vi "Main.vi"() -> ()   [LabVIEW 2014]
doc: "This template is for the Queued Message Handler design pattern.\n\nThe Event Handling Loop generates messages based on user interface actions.\n\nThe Message Handling Loop processes messages generated by the Event Handling Loop, or by other messages. The messages are string values, so new messages can be added easily to the Message Cases case structure in the Message Handling Loop. Each message cluster can also provide an optional value for Message Data, which is a variant that can be converted to whatever message-specific data is required."
uses:
  controls/MHL Data.ctl
  controls/MHL UI Data.ctl
  controls/MHL Status.ctl
  controls/MHL References.ctl
  controls/MHL Configuration.ctl
  support/Boiler System Globals.vi
  support/Message Queue/Message Queue.lvlib
  support/User Event - Stop/User Event - Stop.lvlib
  Boiler/Boiler.lvlib
panel:
  in  "Fuel Control Valve":u32(slide) scale=10.0..75.0
  in  "Stop Boiler":bool
  in  "Light Pilot":bool
  out "Forced Draft Fan":bool
  out "Pilot":bool
  out "Pilot Gas Valve":bool
  out "Primary Fan":bool
  out "Status":string
  in  "Start":bool
  in  "Reset":bool
  in  "Emergency Stop":bool
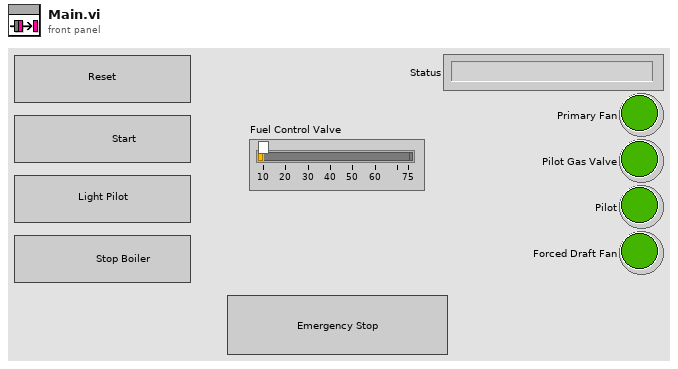
[diagram p1: front panel]
types:
  T1 = typedef "MHL Data.ctl" = cluster{"MHL User Interface Data":T2, "MHL References":T4, "MHL Configuration":T5}
  T2 = typedef "MHL UI Data.ctl" = cluster{"Status":string, "Fuel Control Valve":u32, "Primary Fan":bool, "Pilot Gas Valve":bool, "Pilot":bool, "Forced Draft Fan":bool, "MHL Status":T3}
  T3 = typedef "MHL Status.ctl" = enum16{"Lockout", "Ready", "Pre-Purge", "Pre-Purge Complete", "Pilot On", "Boiler Running", "Shutdown", "Purge"}
  T4 = typedef "MHL References.ctl" = cluster{"Reset Ref":refnum<vi>, "Start Ref":refnum<vi>, "Light Pilot Ref":refnum<vi>, "Stop Boiler Ref":refnum<vi>, "Fuel Control Valve Ref":refnum<vi>}
  T5 = typedef "MHL Configuration.ctl" = cluster{"Fuel Control Valve Maximum":dbl, "Fuel Control Valve Minimum":dbl}
  T6 = typedef "Notifiers.ctl" = cluster{"Handshake":refnum<notifier>, "Flame Level":refnum<notifier>, "Controller Exit":refnum<notifier>, "Boiler Exit":refnum<notifier>}
  T7 = typedef "Message Queue.lvlib/All Message Queues.ctl" = cluster{"MHL":refnum<queue>, "Boiler Controller":refnum<queue>, "Boiler":refnum<queue>}
  T8 = enum32{"invalid app kind", "Development System", "Run Time System", "Student Edition", "Embedded LabVIEW", "Evaluation", "Custom"}
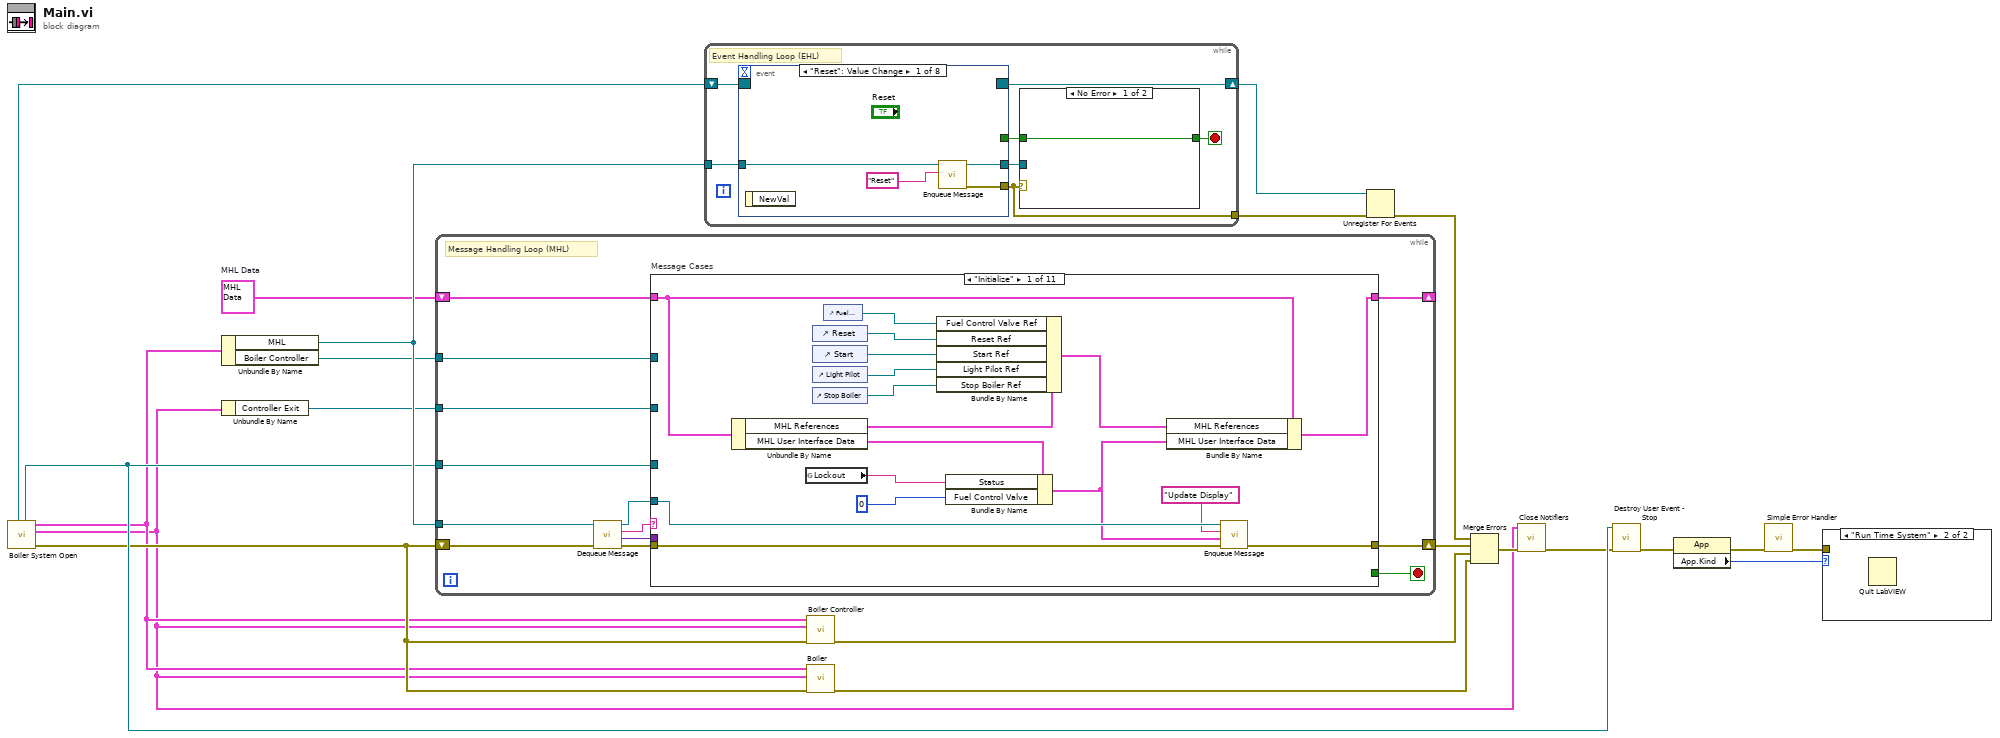
[diagram p0: block diagram]
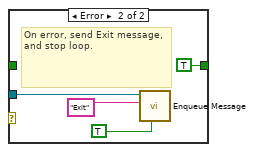
[diagram p3: hidden frame]
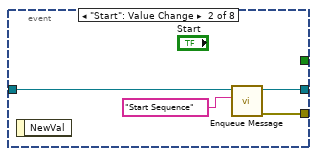
[diagram p4: hidden frame]
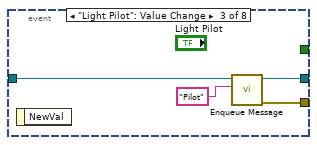
[diagram p5: hidden frame]
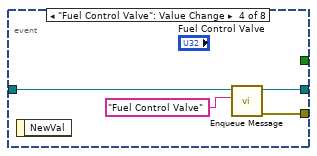
[diagram p6: hidden frame]
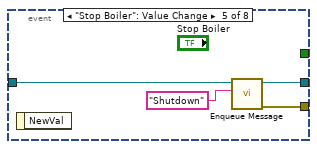
[diagram p7: hidden frame]
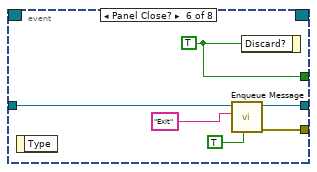
[diagram p8: hidden frame]
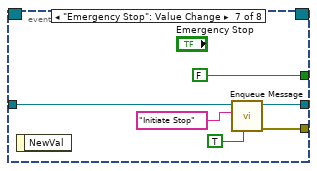
[diagram p9: hidden frame]
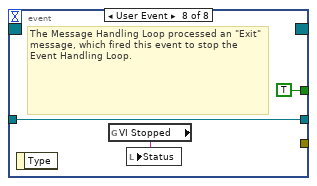
[diagram p10: hidden frame]
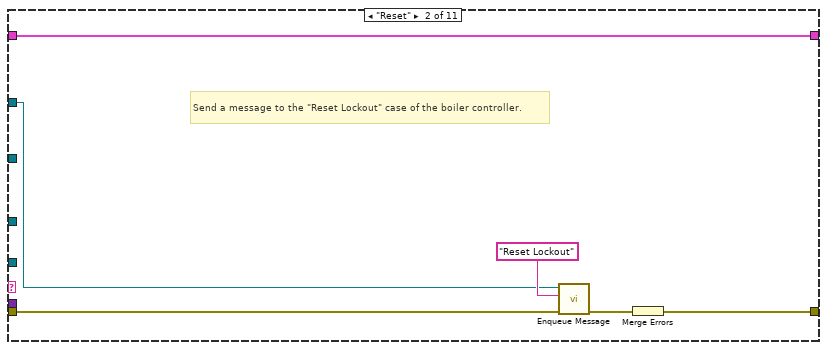
[diagram p11: hidden frame]
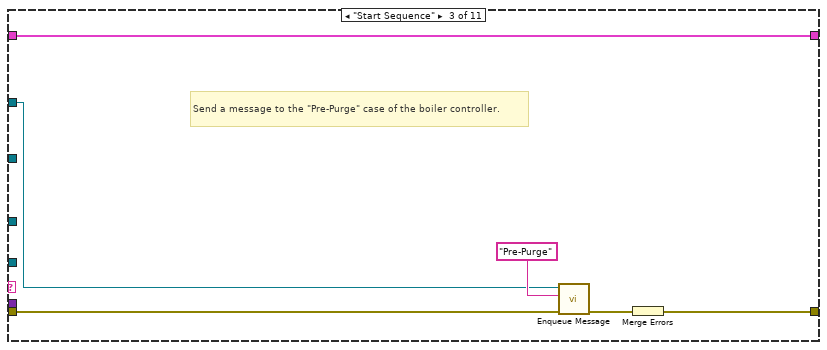
[diagram p12: hidden frame]
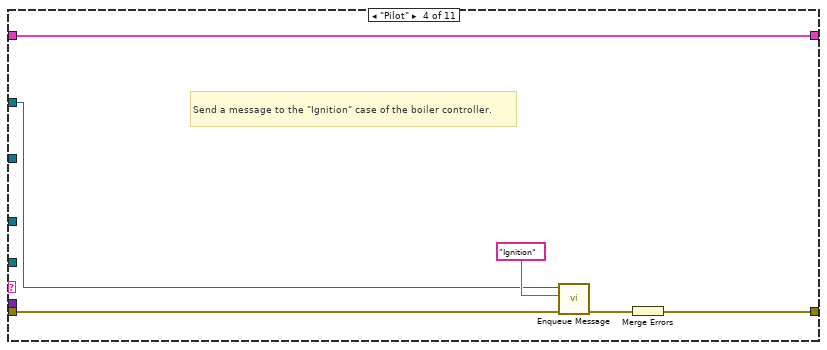
[diagram p13: hidden frame]
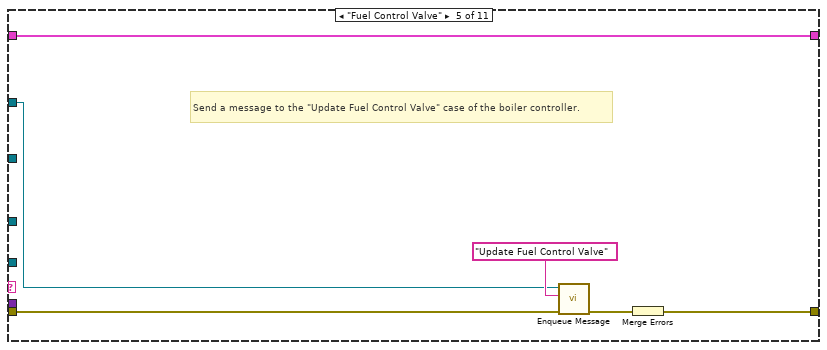
[diagram p14: hidden frame]
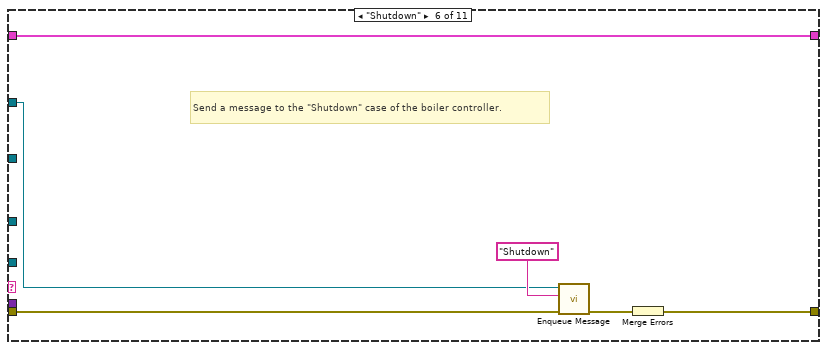
[diagram p15: hidden frame]
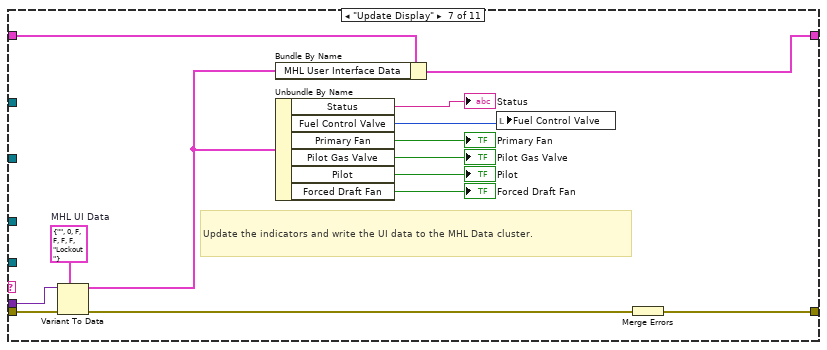
[diagram p16: hidden frame]
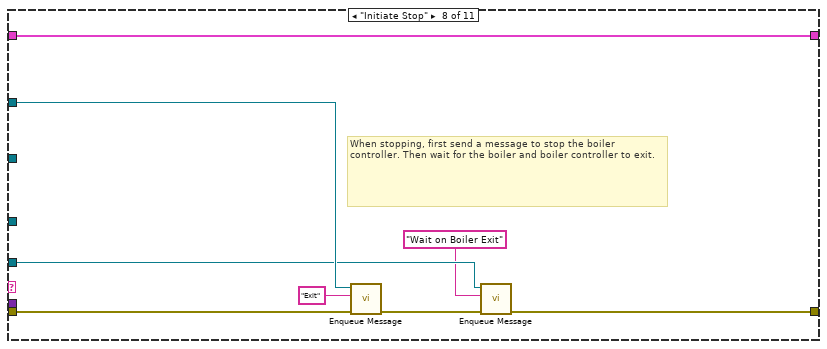
[diagram p17: hidden frame]
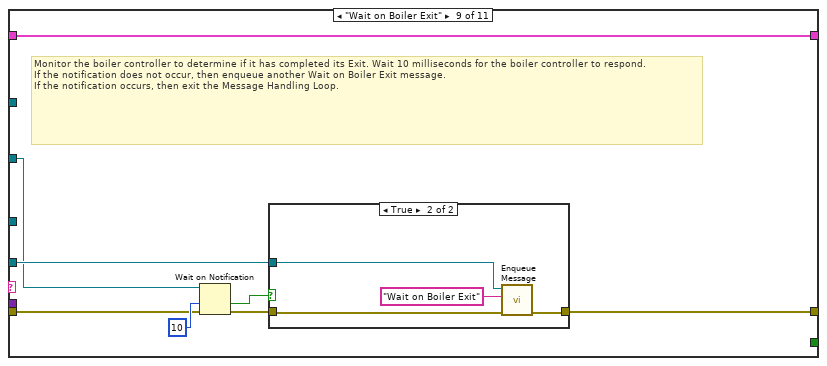
[diagram p18: hidden frame]
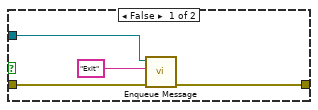
[diagram p19: hidden frame]
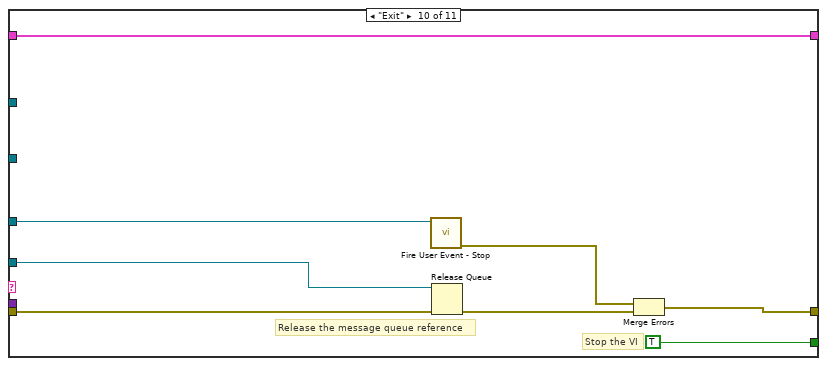
[diagram p20: hidden frame]
diagram:
  w15 = T1 {"MHL User Interface Data"={"Status"="", "Fuel Control Valve"=0, "Primary Fan"=FALSE, "Pilot Gas Valve"=FALSE, "Pilot"=FALSE, "Forced Draft Fan"=FALSE, "MHL Status"=enum."Lockout"}, "MHL References"={"Reset Ref"=refnum, "Start Ref"=refnum, "Light Pilot Ref"=refnum, "Stop Boiler Ref"=refnum, "Fuel Control Valve Ref"=refnum}, "MHL Configuration"={"Fuel Control Valve Maximum"=0.0, "Fuel Control Valve Minimum"=0.0}}  # MHL Data
  n1 = call "Boiler System Open.vi"() -> ("error out"=w6:errorcluster, "Notifiers"=w1:T6, "Message Queues"=w5:T7, "User Event - Stop"=w8:refnum<user-event>, "Stop Event Registration Refnum"=w9:refnum<event-registration>)  [unwired: 7 in]
  n2 = Unbundle By Name(w5) -> ("MHL"=w20:refnum<queue>, "Boiler Controller"=w13:refnum<queue>)
  n3 = Unbundle By Name(w1) -> ("Controller Exit"=w7:refnum<notifier>)
  n4 = while {
    tunnel: w20 -> [w24]
    shift-right: [w33] -> _
    shift-left: w15 -> [w34]
    tunnel: w8 -> [w30]
    shift-right: [w31] -> w21
    shift-left: w6 -> [w29]
    tunnel: w13 -> [w23]
    tunnel: w7 -> [w22]
    stop <- w32 stop-if-true
    # "Message Handling Loop (MHL)"
    n5 = call "Dequeue Message.vi"("error in (no error)"=w29, "Message Queue"=w24) -> ("error out"=w28:errorcluster, "Message Data"=w26:variant, "Message"=w27:string, "dup Message Queue"=w25:refnum<queue>)  [unwired: 6 in]
    n6 = case "Message Cases" shown="\"Initialize\"" w27 {
      selector: w27 -> [_ _ _ _ _ _ _ _ _ _ w131]
      tunnel: w25 -> [w38 _ _ _ _ _ _ w98 w105 w127 _]
      tunnel: w28 -> [w39 w55 w61 w67 w73 w79 w94 w103 w107 w120 _]
      tunnel: [w40 w56 w62 w68 w74 w80 w95 w100 w106 w123 w129] -> w31
      tunnel: w34 -> [w45 w57 w63 w69 w75 w81 w84 w102 w111 w126 w133]
      tunnel: [w44 w57 w63 w69 w75 w81 w82 w102 w111 w126 w133] -> w33
      tunnel: [_ _ _ _ _ _ _ _ _ TRUE _] -> w32
      tunnel: w26 -> [_ _ _ _ _ _ w93 _ _ _ _]
      tunnel: w30 -> [_ _ _ _ _ _ _ _ _ w122 _]
      tunnel: w23 -> [_ w52 w58 w64 w70 w76 _ w99 _ _ _]
      tunnel: w22 -> [_ _ _ _ _ _ _ _ w104 _ _]
      frame "Initialize" {
        n7 = Unbundle By Name(w45) -> ("MHL References"=w43:T4, "MHL User Interface Data"=w42:T2)
        n8 = global read "Boiler System Globals.vi" "Lockout"() -> (w35:string)
        n9 = control-ref of="Reset"() -> (w48:refnum<vi>)
        n10 = control-ref of="Start"() -> (w49:refnum<vi>)
        n11 = control-ref of="Light Pilot"() -> (w50:refnum<vi>)
        n12 = control-ref of="Stop Boiler"() -> (w51:refnum<vi>)
        n13 = control-ref of="Fuel Control Valve"() -> (w47:refnum<vi>)
        n14 = Bundle By Name(cluster=w43, "Fuel Control Valve Ref"=w47, "Reset Ref"=w48, "Start Ref"=w49, "Light Pilot Ref"=w50, "Stop Boiler Ref"=w51) -> (w41:T4)
        n15 = Bundle By Name(cluster=w42, "Status"=w35, "Fuel Control Valve"=u32 0) -> (w37:T2)
        n16 = Bundle By Name(cluster=w45, "MHL References"=w41, "MHL User Interface Data"=w37) -> (w44:T1)
        n17 = call "Enqueue Message.vi"("error in (no error)"=w39, "Message Data"=w37, "Message"="Update Display", "Message Queue"=w38) -> ("error out"=w40:errorcluster)  [unwired: 6 in, 1 out]
      }
      frame "Reset" {
        # "Send a message to the \"Reset Lockout\" case of the boiler controller."
        n18 = call "Enqueue Message.vi"("error in (no error)"=w55, "Message"="Reset Lockout", "Message Queue"=w52) -> ("error out"=w54:errorcluster)  [unwired: 7 in, 1 out]
        n19 = Merge Errors(w54) -> (w56:errorcluster)
      }
      frame "Start Sequence" {
        # "Send a message to the \"Pre-Purge\" case of the boiler controller."
        n20 = call "Enqueue Message.vi"("error in (no error)"=w61, "Message"="Pre-Purge", "Message Queue"=w58) -> ("error out"=w60:errorcluster)  [unwired: 7 in, 1 out]
        n21 = Merge Errors(w60) -> (w62:errorcluster)
      }
      frame "Pilot" {
        # "Send a message to the \"Ignition\" case of the boiler controller."
        n22 = call "Enqueue Message.vi"("error in (no error)"=w67, "Message"="Ignition", "Message Queue"=w64) -> ("error out"=w66:errorcluster)  [unwired: 7 in, 1 out]
        n23 = Merge Errors(w66) -> (w68:errorcluster)
      }
      frame "Fuel Control Valve" {
        # "Send a message to the \"Update Fuel Control Valve\" case of the boiler controller."
        n24 = call "Enqueue Message.vi"("error in (no error)"=w73, "Message"="Update Fuel Control Valve", "Message Queue"=w70) -> ("error out"=w72:errorcluster)  [unwired: 7 in, 1 out]
        n25 = Merge Errors(w72) -> (w74:errorcluster)
      }
      frame "Shutdown" {
        # "Send a message to the \"Shutdown\" case of the boiler controller."
        n26 = call "Enqueue Message.vi"("error in (no error)"=w79, "Message"="Shutdown", "Message Queue"=w76) -> ("error out"=w78:errorcluster)  [unwired: 7 in, 1 out]
        n27 = Merge Errors(w78) -> (w80:errorcluster)
      }
      frame "Update Display" {
        w91 = T2 {"Status"="", "Fuel Control Valve"=0, "Primary Fan"=FALSE, "Pilot Gas Valve"=FALSE, "Pilot"=FALSE, "Forced Draft Fan"=FALSE, "MHL Status"=enum."Lockout"}  # MHL UI Data
        # "Update the indicators and write the UI data to the MHL Data cluster."
        n28 = Variant To Data(error in=w94, type=w91, Variant=w93) -> (data=w83:T2, error out=w92:errorcluster)
        n29 = Bundle By Name(cluster=w84, "MHL User Interface Data"=w83) -> (w82:T1)
        n30 = Unbundle By Name(w83) -> ("Status"=→"Status":string, "Fuel Control Valve"=w89:u32, "Primary Fan"=→"Primary Fan":bool, "Pilot Gas Valve"=→"Pilot Gas Valve":bool, "Pilot"=→"Pilot":bool, "Forced Draft Fan"=→"Forced Draft Fan":bool)
        n31 = local write "Fuel Control Valve"(w89) -> ()
        n32 = Merge Errors(w92) -> (w95:errorcluster)
      }
      frame "Initiate Stop" {
        # "When stopping, first send a message to stop the boiler controller. Then wait for the boiler and boiler controller to exit."
        n33 = call "Enqueue Message.vi"("error in (no error)"=w103, "Message"="Exit", "Message Queue"=w99) -> ("error out"=w101:errorcluster)  [unwired: 7 in, 1 out]
        n34 = call "Enqueue Message.vi"("error in (no error)"=w101, "Message"="Wait on Boiler Exit", "Message Queue"=w98) -> ("error out"=w100:errorcluster)  [unwired: 7 in, 1 out]
      }
      frame "Wait on Boiler Exit" {
        # "Monitor the boiler controller to determine if it has completed its Exit. Wait 10 milliseconds for the boiler controller to respond. \nIf the notification does not occur, then enqueue another Wait on Boiler Exit message.\nIf the notification occurs, then exit the Message Handling Loop."
        n35 = Wait on Notification(notifier=w104, timeout in ms (-1)=10, error in (no error)=w107) -> (timed out?=w109:bool, error out=w108:errorcluster)  [unwired: 1 in, 2 out]
        n36 = case shown="True" w109 {
          tunnel: w108 -> [w115 w119]
          tunnel: w105 -> [w114 w117]
          tunnel: [w112 w118] -> w106
          frame False {
            n37 = call "Enqueue Message.vi"("error in (no error)"=w115, "Message"="Exit", "Message Queue"=w114) -> ("error out"=w112:errorcluster)  [unwired: 7 in, 1 out]
          }
          frame True {
            n38 = call "Enqueue Message.vi"("error in (no error)"=w119, "Message"="Wait on Boiler Exit", "Message Queue"=w117) -> ("error out"=w118:errorcluster)  [unwired: 7 in, 1 out]
          }
        }
      }
      frame "Exit" {
        # "Stop the VI"
        # "Release the message queue reference"
        n39 = call "Fire User Event - Stop.vi"("User Event - Stop"=w122) -> ("error out"=w121:errorcluster)  [unwired: 10 in]
        n40 = Release Queue(queue=w127, error in (no error)=w120) -> (error out=w124:errorcluster)  [unwired: 1 in, 2 out]
        n41 = Merge Errors(w121, w124) -> (w123:errorcluster)
      }
      frame Default {
        # "'Default' case only runs if there is a message that isn't defined in any of the other cases.  Output a programming error."
        n42 = Format Into String(format string="The invalid message string \"%s\" was received in the Message Handling Loop." ("Unknown Message Error Text"), w131) -> (resulting string=w128:string)  [unwired: 2 in, 1 out]
        n43 = call <vilib>:"Error Cluster From Error Code.vi"("error message (\"\")"=w128, "error code (0)"=1) -> ("error out"=w129:errorcluster)  [unwired: 7 in]
      }
    }
  }
  n44 = while {
    tunnel: w20 -> [w140]
    tunnel: [w136] -> w17
    shift-right: [w134] -> w16
    shift-left: w9 -> [w135]
    stop <- w138 stop-if-true
    # "Event Handling Loop (EHL)"
    n45 = event shown="[0] \"Reset\": Value Change" {
      selector: w135 -> [_ _ _ _ _ _ _ _]
      dyn-events: [_ _ _ _ _ _ _ _] -> w134
      timeout: _ -> [_ _ _ _ _ _ _ _]
      tunnel: [_ _ _ _ _ w171 FALSE ("Discard?") TRUE ("Discard?")] -> w139
      tunnel: w140 -> [w149 w153 w157 w161 w165 w170 w177 w180]
      tunnel: [w148 w151 w155 w159 w163 w169 w176 _] -> w136
      tunnel: [w147 w152 w156 w160 w164 w168 w174 w180] -> w137
      event "Reset": Value Change {
        n46 = event-data() -> ()  [unwired: 1 in, 1 out]
        n47 = call "Enqueue Message.vi"("Message"="Reset", "Message Queue"=w149) -> ("error out"=w148:errorcluster, "dup Message Queue"=w147:refnum<queue>)  [unwired: 8 in]
      }
      event "Start": Value Change {
        n48 = event-data() -> ()  [unwired: 1 in, 1 out]
        n49 = call "Enqueue Message.vi"("Message"="Start Sequence", "Message Queue"=w153) -> ("error out"=w151:errorcluster, "dup Message Queue"=w152:refnum<queue>)  [unwired: 8 in]
      }
      event "Light Pilot": Value Change {
        n50 = event-data() -> ()  [unwired: 1 in, 1 out]
        n51 = call "Enqueue Message.vi"("Message"="Pilot", "Message Queue"=w157) -> ("error out"=w155:errorcluster, "dup Message Queue"=w156:refnum<queue>)  [unwired: 8 in]
      }
      event "Fuel Control Valve": Value Change {
        n52 = event-data() -> ()  [unwired: 1 in, 1 out]
        n53 = call "Enqueue Message.vi"("Message"="Fuel Control Valve", "Message Queue"=w161) -> ("error out"=w159:errorcluster, "dup Message Queue"=w160:refnum<queue>)  [unwired: 8 in]
      }
      event "Stop Boiler": Value Change {
        n54 = event-data() -> ()  [unwired: 1 in, 1 out]
        n55 = call "Enqueue Message.vi"("Message"="Shutdown", "Message Queue"=w165) -> ("error out"=w163:errorcluster, "dup Message Queue"=w164:refnum<queue>)  [unwired: 8 in]
      }
      event Panel Close? {
        w171 = TRUE ("Discard?")
        n56 = event-data() -> ()  [unwired: 1 in, 1 out]
        n57 = call "Enqueue Message.vi"("Priority Message? (F)"=TRUE, "Message"="Exit", "Message Queue"=w170) -> ("error out"=w169:errorcluster, "dup Message Queue"=w168:refnum<queue>)  [unwired: 7 in]
        n58 = event-data("Discard?"=w171) -> ()  [unwired: 1 in, 1 out]
      }
      event "Emergency Stop": Value Change {
        n59 = event-data() -> ()  [unwired: 1 in, 1 out]
        n60 = call "Enqueue Message.vi"("Priority Message? (F)"=TRUE, "Message"="Initiate Stop", "Message Queue"=w177) -> ("error out"=w176:errorcluster, "dup Message Queue"=w174:refnum<queue>)  [unwired: 7 in]
      }
      event User Event {
        # "The Message Handling Loop processed an \"Exit\" message, which fired this event to stop the Event Handling Loop."
        n61 = event-data() -> ()  [unwired: 1 in, 1 out]
        n62 = global read "Boiler System Globals.vi" "VI Stopped"() -> (w178:string)
        n63 = local write "Status"(w178) -> ()
      }
    }
    n64 = case shown="No Error" w136 {
      tunnel: [w141 TRUE ("Discard?")] -> w138
      tunnel: w139 -> [w141 _]
      tunnel: w137 -> [_ w144]
      frame No Error {
      }
      frame Error {
        # "On error, send Exit message, and stop loop."
        n65 = call "Enqueue Message.vi"("Priority Message? (F)"=TRUE, "Message"="Exit", "Message Queue"=w144) -> ()  [unwired: 7 in, 2 out]
      }
    }
  }
  n66 = call "Boiler Controller.vi"("error in"=w6, "Notifiers"=w1, "Message Queues"=w5) -> ("error out"=w14:errorcluster)  [unwired: 8 in]
  n67 = call "Boiler.vi"("error in"=w6, "Notifiers"=w1, "Message Queues"=w5) -> ("error out"=w4:errorcluster)  [unwired: 8 in]
  n68 = Unregister For Events(event registration refnum=w16, error in=w17) -> (error out=w18:errorcluster)
  n69 = Merge Errors(w18, w21, w14, w4) -> (w3:errorcluster)
  n70 = call "Close Notifiers.vi"("error in"=w3, "Notifiers"=w1) -> ("error out"=w2:errorcluster)  [unwired: 9 in]
  n71 = call "Destroy User Event - Stop.vi"("error in (no error)"=w2, "User Event - Stop"=w8) -> ("error out"=w19:errorcluster)  [unwired: 9 in]
  n72 = property class="App"(error in=w19) -> (error out=w12:errorcluster, "App.Kind"=w11:T8)  [unwired: 1 in, 1 out]
  n73 = call <vilib>:"Simple Error Handler.vi"("error in (no error)"=w12) -> ("error out"=w10:errorcluster)  [unwired: 4 in, 4 out]
  n74 = case shown="\"Run Time System\"" w11 {
    tunnel: w10 -> [_ _]
    frame Default {
    }
    frame "Run Time System" {
      n75 = Quit LabVIEW() -> ()  [unwired: 1 in]
    }
  }
